vi "Marker Calibration.vi"(8 "Marker Location":dbl[](array[numeric]), 11 "Match":T1(array[cluster])) -> (0 "Encoder Setpoint":i32[](array[numeric]), 1 "Joint Coordinates (rad) (new)":dbl[](array[numeric]), 3 "Joint Coordinates (rad) (old)":dbl[](array[numeric]))   [LabVIEW 2019]
panel:
  out "task (new)":dbl[](array[numeric])
  out "task (old)":dbl[](array[numeric])
  out "Theta_0":dbl
  out "Theta_1":dbl
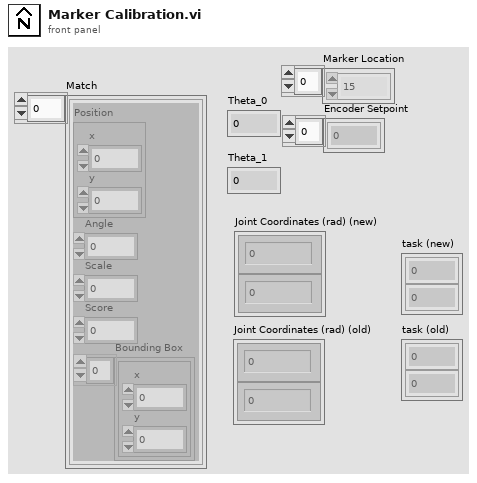
[diagram p1: front panel]
types:
  T1 = cluster{"Position":cluster{"x":sgl, "y":sgl}, "Angle":sgl, "Scale":sgl, "Score":sgl, "Bounding Box":cluster{"x":sgl, "y":sgl}[]}[]
  T2 = cluster{"Position":cluster{"x":sgl, "y":sgl}, "Angle":sgl, "Scale":sgl, "Score":sgl, "Bounding Box":cluster{"x":sgl, "y":sgl}[]}
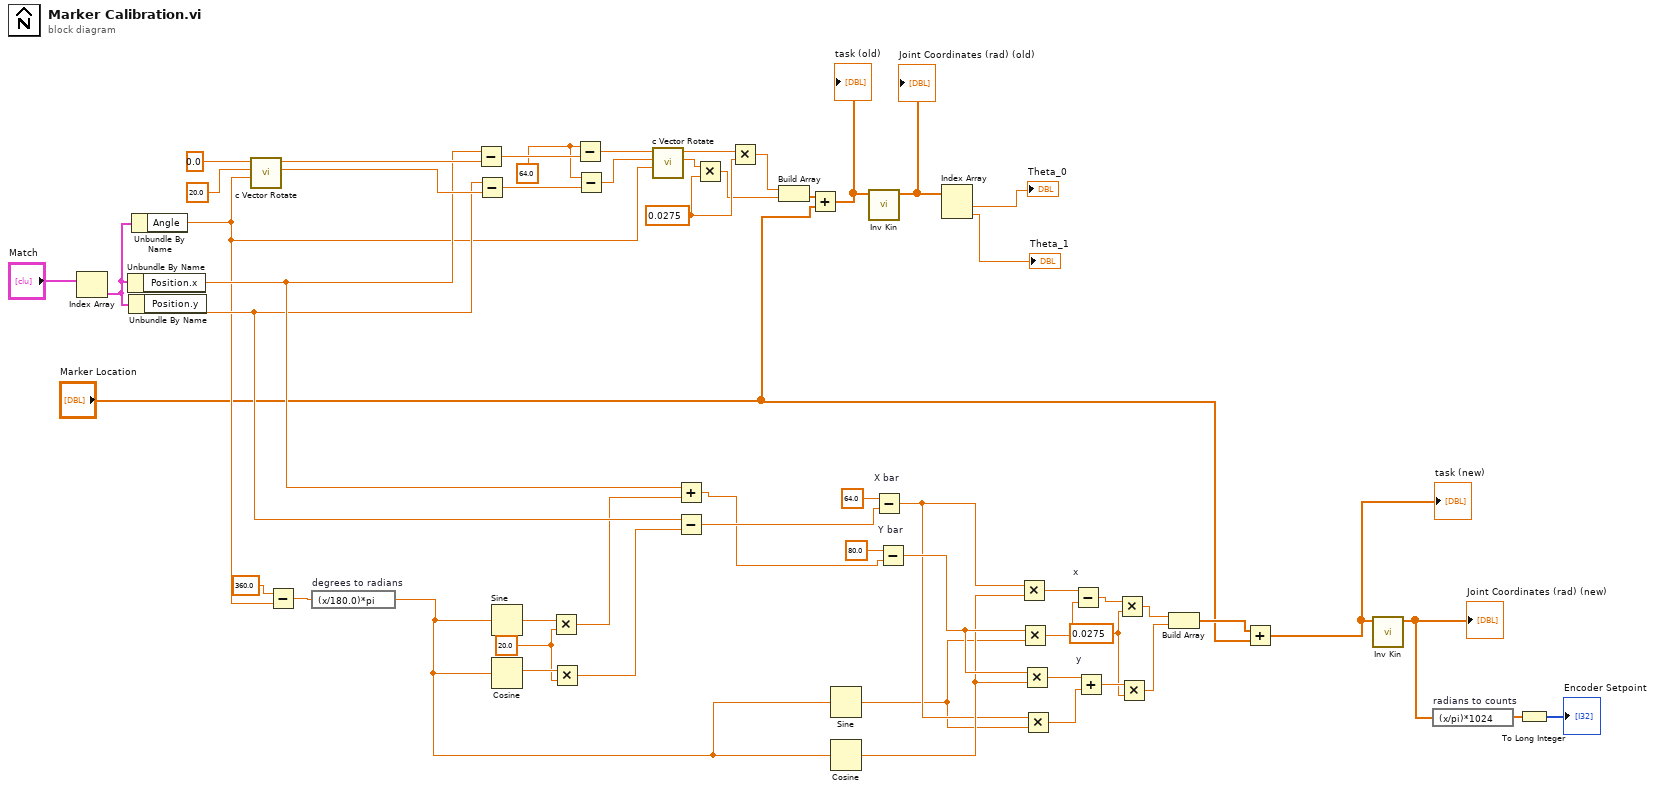
[diagram p0: block diagram]
diagram:
  w17 = 0.0275 ("y")
  w34 = sgl 20.0 ("y")
  w55 = 0.0275 ("y")
  w50 = 64.0 ("y")
  n1 = Index Array(array="Match") -> (element=w4:T2)  [unwired: 1 in]
  n2 = Unbundle By Name(w4) -> ("Position.x"=w40:sgl)
  n3 = Unbundle By Name(w4) -> ("Position.y"=w39:sgl)
  n4 = Unbundle By Name(w4) -> ("Angle"=w38:sgl)
  n5 = call "c Vector Rotate.vi"("Angle"=w38, "Y"=20.0, "X"=0.0) -> ("New Y"=w47:dbl, "New X"=w46:dbl)  [unwired: 7 in]
  n6 = Subtract(x=sgl 360.0, y=w38) -> (x-y=w16:sgl)
  n7 = expression code="(x/180.0)*pi" "degrees to radians"(w16) -> (w15:sgl)
  n8 = Subtract(x=w40, y=w46) -> (x-y=w51:dbl)
  n9 = Subtract(x=w39, y=w47) -> (x-y=w52:dbl)
  n10 = Sine(x=w15) -> (sin(x)=w36:sgl)
  n11 = Cosine(x=w15) -> (cos(x)=w35:sgl)
  n12 = Multiply(x=w36, y=w34) -> (x*y=w33:sgl)
  n13 = Multiply(x=w35, y=w34) -> (x*y=w32:sgl)
  n14 = Subtract(x=w50, y=w51) -> (x-y=w48:dbl)
  n15 = Subtract(x=w50, y=w52) -> (x-y=w49:dbl)
  n16 = call "c Vector Rotate.vi"("Angle"=w38, "Y"=w49, "X"=w48) -> ("New Y"=w53:dbl, "New X"=w54:dbl)  [unwired: 7 in]
  n17 = Add(x=w40, y=w33) -> (x+y=w28:sgl)
  n18 = Subtract(x=w39, y=w32) -> (x-y=w29:sgl)
  n19 = Multiply(x=w53, y=w55) -> (x*y=w14:dbl)
  n20 = Multiply(x=w54, y=w55) -> (x*y=w13:dbl)
  n21 = Build Array(w13, w14) -> (w12:dbl[])
  n22 = Add(x=w12, y="Marker Location") -> (x+y=w11:dbl[])
  "task (old)" <- w11
  n23 = Sine(x=w15) -> (sin(x)=w20:sgl)
  n24 = Cosine(x=w15) -> (cos(x)=w22:sgl)
  n25 = call "Inv Kin.vi"("Task Coordinates (cm)"=w11) -> ("Joint Coordinates (rad)"=w43:dbl[])  [unwired: 10 in]
  "Joint Coordinates (rad) (old)" <- w43
  n26 = Subtract "X bar"(x=64.0, y=w29) -> (x-y=w21:dbl)
  n27 = Subtract "Y bar"(x=80.0, y=w28) -> (x-y=w23:dbl)
  n28 = Index Array(array=w43) -> (element #1=→"Theta_0":dbl, element #2=→"Theta_1":dbl)  [unwired: 2 in]
  n29 = Multiply(x=w21, y=w22) -> (x*y=w27:dbl)
  n30 = Multiply(x=w23, y=w20) -> (x*y=w26:dbl)
  n31 = Multiply(x=w23, y=w22) -> (x*y=w25:dbl)
  n32 = Multiply(x=w21, y=w20) -> (x*y=w24:dbl)
  n33 = Subtract "x"(x=w27, y=w26) -> (x-y=w18:dbl)
  n34 = Add "y"(x=w25, y=w24) -> (x+y=w19:dbl)
  n35 = Multiply(x=w18, y=w17) -> (x*y=w10:dbl)
  n36 = Multiply(x=w19, y=w17) -> (x*y=w9:dbl)
  n37 = Build Array(w10, w9) -> (w8:dbl[])
  n38 = Add(x=w8, y="Marker Location") -> (x+y=w6:dbl[])
  "task (new)" <- w6
  n39 = call "Inv Kin.vi"("Task Coordinates (cm)"=w6) -> ("Joint Coordinates (rad)"=w3:dbl[])  [unwired: 10 in]
  "Joint Coordinates (rad) (new)" <- w3
  n40 = expression code="(x/pi)*1024" "radians to counts"(w3) -> (w2:dbl[])
  n41 = To Long Integer(number=w2) -> (32bit integer=→"Encoder Setpoint":i32[])
